vi "get Displacement.vi"(11 "Motion in":refnum<class "Motion.lvclass">) -> (3 "Displacement":refnum<class "Vector 2D.lvclass">)   [LabVIEW 2015, in "Motion.lvclass"]
uses:
  Motion.lvclass
  Vector 2D/Vector 2D.lvclass
  Motion.lvclass/Motion.ctl
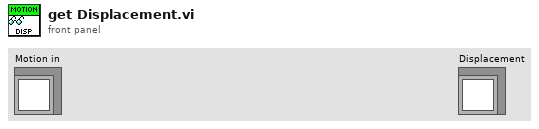
[diagram p1: front panel]
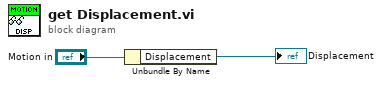
[diagram p0: block diagram]
diagram:
  n1 = Unbundle By Name("Motion in") -> ("Displacement"=→"Displacement":refnum<class "Vector 2D.lvclass">)
